vi "Read Backpressure Subscriber.vi"(8 "error in (no error)":errorcluster, 11 "CIF_CIPC_Chn in":refnum<class "CIF_CIPC_Chn.lvclass">) -> (0 "error out":errorcluster, 2 "Backpressure Subscriber":string, 3 "CIF_CIPC_Chn out":refnum<class "CIF_CIPC_Chn.lvclass">)   [LabVIEW 2021, in "CIF_CIPC_Chn.lvclass"]
uses:
  CIF_CIPC_Chn.lvclass
  CIF_CIPC_Chn.lvclass/CIF_CIPC_Chn.ctl
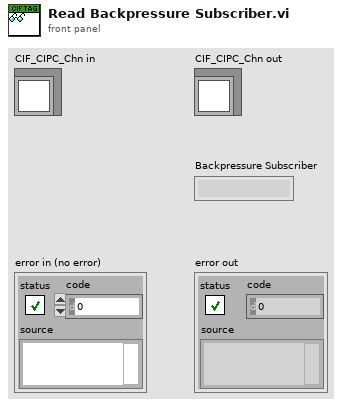
[diagram p1: front panel]
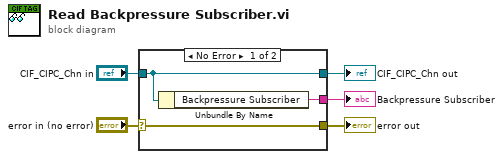
[diagram p0: block diagram]
diagram:
  n1 = case shown="No Error" "error in (no error)" {
    selector: "error in (no error)" -> [w8 w9]
    tunnel: [w8 w9] -> w4
    tunnel: [w7 w10] -> w2
    tunnel: "CIF_CIPC_Chn in" -> [w7 w10]
    tunnel: [w6 _] -> w1
    frame No Error {
      n2 = Unbundle By Name(w7) -> ("Backpressure Subscriber"=w6:string)
    }
    frame Error {
    }
  }
  "error out" <- w4
  "CIF_CIPC_Chn out" <- w2
  "Backpressure Subscriber" <- w1
